vi "URAPI_GoSub.vi"(2 "Subroutine Name":string="Sub1", 3 "URAPI Script":T1) -> (1 "URAPI Script out":T1)   [LabVIEW 2012]
uses:
  <userlib>/BotSpeak/VIs/Direct/URAPI_Control.ctl
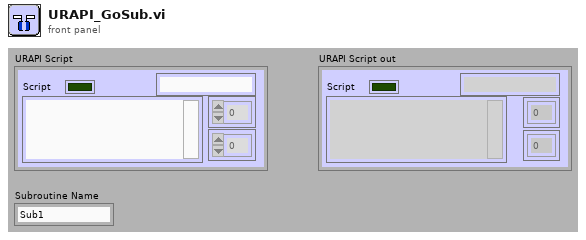
[diagram p1: front panel]
types:
  T1 = typedef "URAPI_Control.ctl" = cluster{"Script":string, "Whiles":u8[], "Ifs":u8[], "Supress Err":bool, "Errors":string}
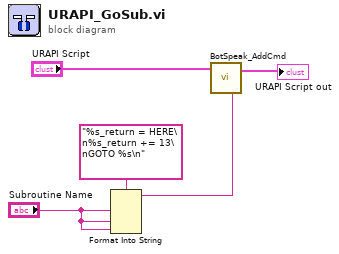
[diagram p0: block diagram]
diagram:
  n1 = Format Into String(format string="%s_return = HERE\n%s_return += 13\nGOTO %s\n" ("String"), "Subroutine Name", "Subroutine Name", "Subroutine Name") -> (resulting string=w4:string)  [unwired: 2 in, 1 out]
  n2 = call <userlib>:"BotSpeak_AddCmd.vi"("String"=w4, "URAPI Script"="URAPI Script") -> ("URAPI Script out"=→"URAPI Script out":T1)  [unwired: 1 in]
